vi "rs232.vi"() -> ()   [LabVIEW 2023]
uses:
  <vilib>/Instr/_visa.llb/VISA Configure Serial Port (Instr).vi
panel:
  in  "stop":bool
  out "String":string
  in  "VISA resource name":refnum<visa-resource-name>
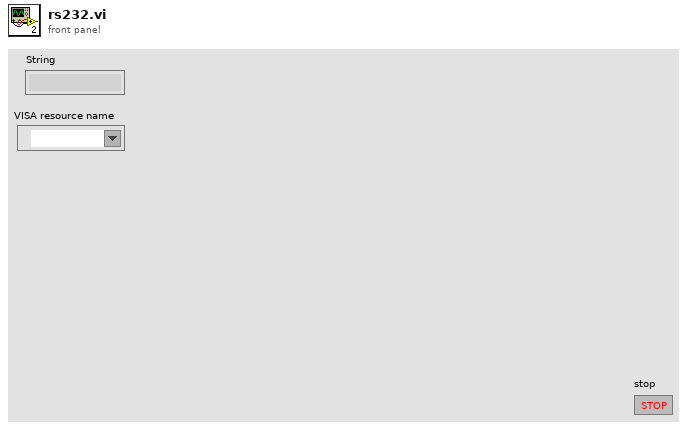
[diagram p1: front panel]
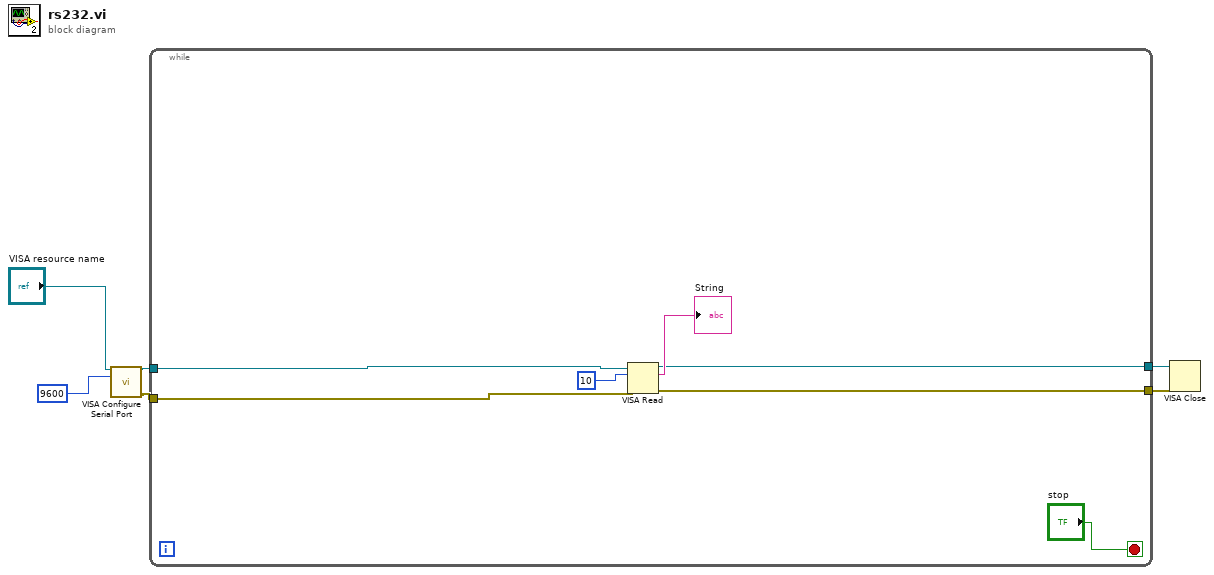
[diagram p0: block diagram]
diagram:
  n1 = call-poly "VISA Configure Serial Port"("VISA resource name"="VISA resource name", "baud rate (9600)"=9600) -> ("VISA resource name out"=w4:refnum<visa-resource-name>, "error out"=w3:errorcluster)  [unwired: 12 in]
  n2 = while {
    tunnel: w4 -> [w8]
    tunnel: w3 -> [w11]
    tunnel: [w10] -> w2
    tunnel: [w9] -> w1
    stop <- "stop" stop-if-true
    n3 = VISA Read(VISA resource name=w8, byte count=10, error in (no error)=w11) -> (VISA resource name out=w9:refnum<visa-resource-name>, read buffer=→"String":string, error out=w10:errorcluster)  [unwired: 1 out]
  }
  n4 = VISA Close(VISA resource name=w1, error in (no error)=w2) -> ()  [unwired: 1 out]
